vi "Fetch Waveform.vi"(8 "Error In":errorcluster, 10 "Channel":u8, 11 "reference in":refnum<class "Scope Base.lvclass">) -> (0 "Error Out":errorcluster, 3 "reference out":refnum<class "Scope Base.lvclass">)   [LabVIEW 2023]
uses:
  Scope Base.lvclass
  Interfaces/IConfigure/IConfigure.lvclass
  Instrument Base/Instrument Base.lvclass
  D:/git/HAL/HAL GOOP4/Instrument Base/Instrument Base.lvclass
  D:/git/HAL/HAL GOOP4/Interfaces/IInstrument Base/IInstrument Base.lvclass
  D:/git/HAL/HAL GOOP4/Scope/Scope Base/Scope Base.lvclass
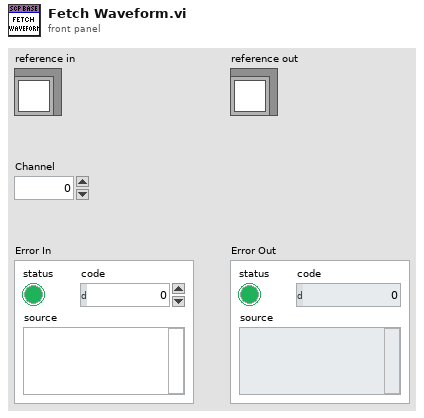
[diagram p1: front panel]
types:
  T1 = typedef "Scope Base.lvlib/Scope Base.lvclass/ObjectAttributes.ctl" = cluster{"Last Waveforms":map{u8, waveform(dbl)}}
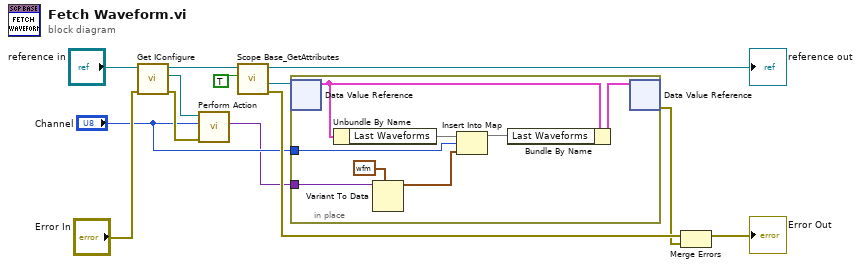
[diagram p0: block diagram]
diagram:
  n1 = call "Get IConfigure.vi"("Error In"="Error In", "reference in"="reference in") -> ("Error Out"=w5:errorcluster, "IConfigure"=w4:refnum<class "IConfigure.lvclass">, "reference out"=w7:refnum<class "Scope Base.lvclass">)  [unwired: 7 in]
  n2 = call-dynamic "Perform Action.vi"("Error In"=w5, "Input"="Channel", "object in"=w4) -> ("Output"=w2:variant)  [unwired: 6 in, 2 out]
  n3 = call "Scope Base_GetAttributes.vi"("OnlyGetDvrReference(False)"=TRUE, "reference in"=w7) -> ("Error Out"=w10:errorcluster, "DataRef"=w11:refnum<data-value>, "reference out"=→"reference out":refnum<class "Scope Base.lvclass">)  [unwired: 6 in, 1 out]
  n4 = in-place {
    in-place-border: "Channel" -> [w17]
    in-place-border: w2 -> [w16]
    n5 = in-place-dvr #1(w11) -> (w20:T1)  [unwired: 1 out]
    n6 = Unbundle By Name(w20) -> ("Last Waveforms"=w19:map{u8, waveform(dbl)})
    n7 = Variant To Data(type=waveform(dbl) {"t0"=timestamp(0 s since 1904-01-01), "dt"=1.0, "Y"=[]} ("Waveform"), Variant=w16) -> (data=w15:waveform(dbl))  [unwired: 1 in, 1 out]
    n8 = Insert Into Map(map in=w19, key=w17, value=w15) -> (map out=w18:map{u8, waveform(dbl)})  [unwired: 2 out]
    n9 = Bundle By Name(cluster=w20, "Last Waveforms"=w18) -> (w21:T1)
    n10 = in-place-dvr #1(w21) -> (w9:errorcluster)  [unwired: 1 out]
  }
  n11 = Merge Errors(w10, w9) -> (→"Error Out":errorcluster)
